vi "Catch Nested Value Update.vi"(8 "error in (no error)":errorcluster, 10 "Nested Value Update Msg":refnum<class "Nested Value Update Msg.lvclass">, 11 "SimpleViewModel In":refnum<class "SimpleViewModel.lvclass">) -> (0 "error out":errorcluster, 3 "SimpleViewModel Out":refnum<class "SimpleViewModel.lvclass">)   [LabVIEW 2015, in "MVAExamples.lvlib" / "SimpleViewModel.lvclass"]
doc: "<License>\nCopyright © 2017 Composed Systems, LLC | All rights reserved\nwww.composed.io\n\nAuthor: Ethan Stern <ethan.stern@composed.io>\n\nThis software is provided \"AS IS\" WITHOUT WARRANTIES, either express or implied, AND IS FOR EDUCATIONAL PURPOSES ONLY.\n</License>"
uses:
  SimpleViewModel.lvclass
  Framework/IViewable/IViewable Messages/Catch Nested Value Change Msg/Nested Value Update Msg.lvclass
  Framework/IViewable/IViewable Messages/Catch Nested Value Change Msg/Nested Value Update Msg.lvclass/Nested Value Update Msg.ctl
  <vilib>/ActorFramework/Actor/Actor.lvclass/Actor.ctl
  <vilib>/ActorFramework/Message Enqueuer/Message Enqueuer.lvclass/Message Enqueuer.ctl
  Framework/IViewModel/IViewModel/IViewModel.lvclass/IViewModel.ctl
  Framework/IMediator/PublishRequest/PublishRequest.lvclass/PublishRequest.ctl
  Framework/AbstractMessages/PreAddressedMsg/PreAddressedMsg.lvclass/PreAddressedMsg.ctl
  Framework/IMediator/IMediator Messages/Publish Msg/Publish Msg.lvclass/Publish Msg.ctl
  ExampleSimpleRootModel Messages/Execute State Msg/Execute State Msg.lvclass/Execute State Msg.ctl
  Framework/IViewable/IViewable Messages/Catch Nested Value Change Msg/Accessors/Read Datum Name.vi
  Framework/IViewable/IViewable Messages/Catch Nested Value Change Msg/Accessors/Read Value.vi
  Framework/IMediator/IMediator Messages/Publish Msg/Send Pre-Addressed Publish.vi
  Framework/IObserver/IObserver/Read Unique ID.vi
  Framework/IMediator/PublishRequest/Pack Publish Request.vi
  <vilib>/ActorFramework/Message Enqueuer/Enqueue.vi
  Framework/AbstractMessages/PreAddressedMsg/Read Return Address.vi
  <vilib>/ActorFramework/Actor/Read Self Enqueuer.vi
  <vilib>/ActorFramework/Message Enqueuer/Init from Existing Queue.vi
  <vilib>/ActorFramework/Message Priority Queue/Priority Enqueue.vi
  <vilib>/ActorFramework/Message Enqueuer/Message Enqueuer.lvclass
  Framework/IMediator/PublishRequest/PublishRequest.lvclass
  ExampleSimpleRootModel Messages/Execute State Msg/Execute State Msg.lvclass
  Framework/IViewModel/IViewModel/IViewModel.lvclass
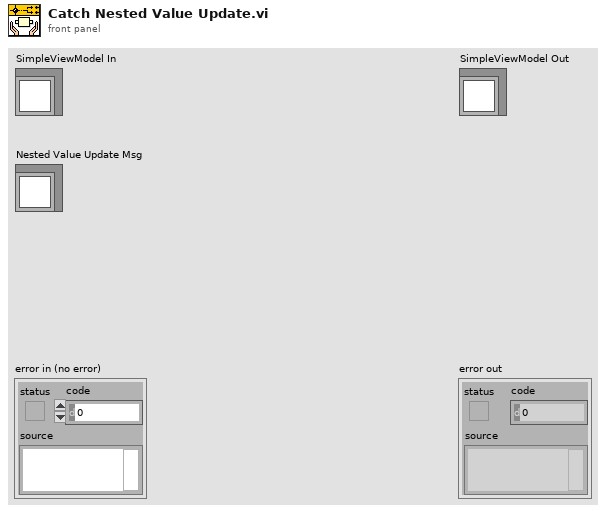
[diagram p1: front panel]
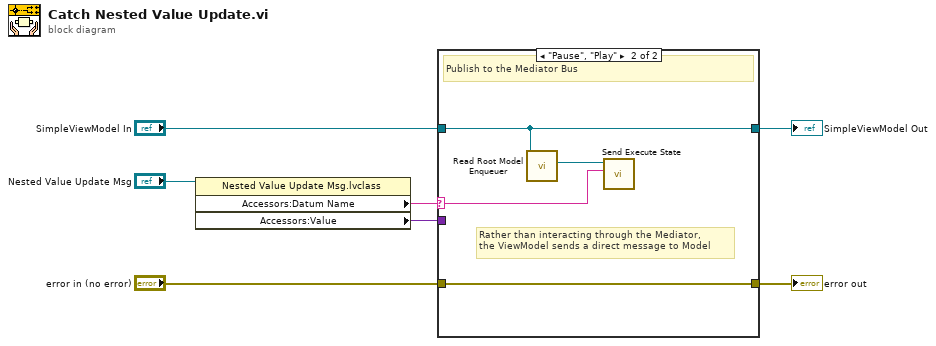
[diagram p0: block diagram]
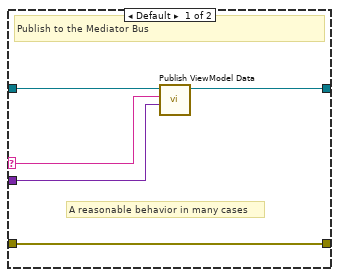
[diagram p2: hidden frame]
diagram:
  n1 = property class="Nested Value Update Msg.lvclass"(reference="Nested Value Update Msg") -> ("Accessors:Datum Name"=w3:string, "Accessors:Value"=w4:variant)  [unwired: 1 in, 2 out]
  n2 = case shown="\"Pause\", \"Play\"" w3 {
    selector: w3 -> [w9 w13]
    tunnel: "SimpleViewModel In" -> [w12 w14]
    tunnel: [w11 w14] -> w6
    tunnel: w4 -> [w10 _]
    tunnel: "error in (no error)" -> [w8 w16]
    tunnel: [w8 w16] -> w1
    frame Default {
      # "A reasonable behavior in many cases"
      # "Publish to the Mediator Bus"
      n3 = call "Publish ViewModel Data.vi"("Data to Publish"=w10, "Datum Name"=w9, "IViewModel In"=w12) -> ("IViewModel Out"=w11:refnum<class "SimpleViewModel.lvclass">)  [unwired: 7 in, 1 out]
    }
    frame "Pause", "Play" {
      # "Rather than interacting through the Mediator,\nthe ViewModel sends a direct message to Model"
      # "Publish to the Mediator Bus"
      n4 = call "Read Root Model Enqueuer.vi"("IViewModel In"=w14) -> ("Model Enqueuer"=w15:refnum<class "Message Enqueuer.lvclass">)  [unwired: 10 in]
      n5 = call "Send Execute State.vi"("State"=w13, "Message Enqueuer"=w15) -> ()  [unwired: 8 in, 2 out]
    }
  }
  "error out" <- w1
  "SimpleViewModel Out" <- w6
